vi "borrar.vi"() -> ()   [LabVIEW 2013]
uses:
  <vilib>/Platform/TimedLoop/XDataNode/timing_clust.ctl
  <vilib>/Platform/TimedLoop/XDataNode/nitl_modes.ctl
  <vilib>/Platform/TimedLoop/XDataNode/wakeup.ctl
  <vilib>/addons/database/Connection.llb/DB Tools Open Connec (Path).vi
  <vilib>/platform/TimedLoop/XDataNode/XDataNode.xnode
  <vilib>/addons/database/_DB Variant To Data/Database Variant To Data.xnode
  <vilib>/Platform/TimedLoop/XDataNode/XDNodeRunTimeDep.lvlib
  <vilib>/addons/database/NI_Database_API.lvlib
panel:
  in  "Menu Ring 2":u16(ring) items=["prueba1", "prueba2", "prueba3", "prueba5"]
  in  "Menu Ring":u16(ring) items=["fallo1", "fallo2", "fallo3"]
  out "data 3":string[](array[string])
  out "data 2":string[](array[string])
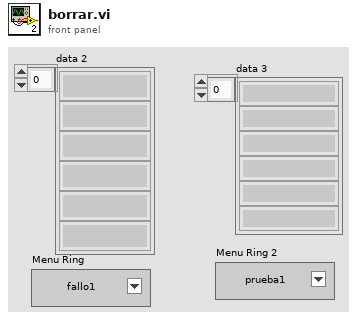
[diagram p1: front panel]
types:
  T1 = typedef "XDNodeRunTimeDep.lvlib/timing_clust.ctl" = cluster{"Expected End [f-1]":u64, "Actual End [f-1]":u64, "Finished Late? [f-1]":bool, "Expected End [i-1]":u64, "Actual End [i-1]":u64, "Finished Late? [i-1]":bool, "Expected Start [i]":u64, "Actual Start [i]":u64, "Expected Start [f]":u64, "Actual Start [f]":u64, "Source Name":string, "Structure Name":string, "Period":i64, "Deadline":i64, "Offset":i64, "Start":i64, "Priority":i32, "Timeout":i32, "Mode":T2, "Wakeup Reason":T3, "Error":errorcluster, "Source Type":string, "Secondary Source Type":string, "Global End Time":u64, "Global Start Time":u64, "Frame Duration":u64, "Iteration Duration":u64, "Assigned CPU":i32, "I/O Scan Engine Mode":u32}
  T2 = typedef "XDNodeRunTimeDep.lvlib/nitl_modes.ctl" = enum32{"No Change", "Process missed periods, maintain original phase", "Discard missed periods, maintain original phase", "Process missed periods, ignore original phase", "Discard missed periods, ignore original phase"}
  T3 = typedef "XDNodeRunTimeDep.lvlib/wakeup.ctl" = enum32{"Normal", "Aborted", "Asynchronous wakeup", "Timing source error", "Timed loop error", "Timeout"}
  T4 = typedef "NI_Database_API.lvlib/Conn ObjectReference.ctl" = refnum<k1>
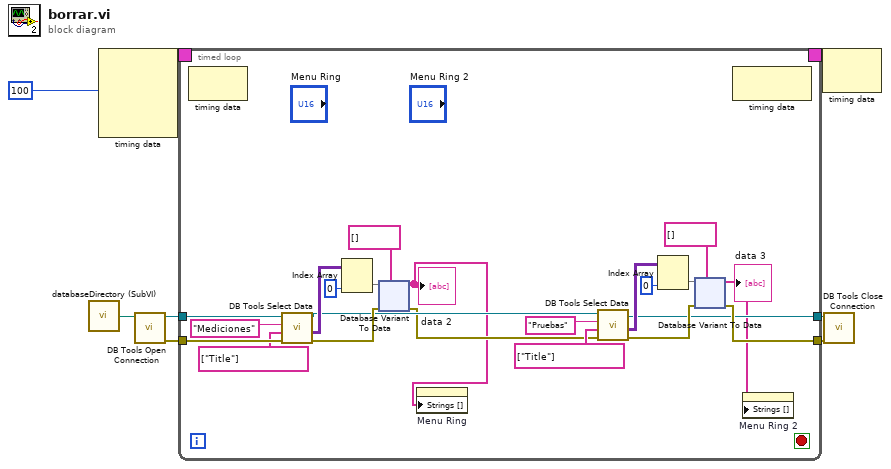
[diagram p0: block diagram]
diagram:
  n1 = call "databaseDirectory (SubVI).vi"() -> ("Application Directory"=w5:path)  [unwired: 1 in]
  n2 = node-c288(i64 100 ("Period")) -> (w8:T1)  [unwired: 3 in]
  n3 = call-poly <vilib>:"DB Tools Open Connection.vi"("connection information"=w5) -> ("error out"=w3:errorcluster, "connection reference"=w4:T4)  [unwired: 7 in]
  n4 = timed-loop {
    timing: w8 -> [_]
    timing-out: [_] -> w7
    tunnel: w4 -> [w30]
    tunnel: w3 -> [w29]
    tunnel: [w12] -> w2
    tunnel: [w11] -> w1
    stop <- _ stop-if-true
    n5 = node-c288() -> ()  [unwired: 1 in, 1 out]
    n6 = call <vilib>:"DB Tools Select Data.vi"("error in (no error)"=w29, "columns"=string[] ["Title"], "table"="Mediciones", "connection reference"=w30) -> ("error out"=w22:errorcluster, "data"=w25:variant[][], "connection reference out"=w14:T4)  [unwired: 2 in]
    n7 = Index Array(array=w25, index (col)=0 ("index")) -> (element=w24:variant[])  [unwired: 1 in]
    n8 = xnode "Database Variant To Data"("database variant"=w24, "error in (no error)"=w22, "type"=string[] []) -> ("data"=w10:string[], "error out"=w13:errorcluster)
    "data 2" <- w10
    n9 = property on="Menu Ring" class="Ring (strict)"("Strings []"=w10) -> ()  [unwired: 2 in, 2 out]
    n10 = call <vilib>:"DB Tools Select Data.vi"("error in (no error)"=w13, "columns"=string[] ["Title"], "table"="Pruebas", "connection reference"=w14) -> ("error out"=w21:errorcluster, "data"=w18:variant[][], "connection reference out"=w11:T4)  [unwired: 2 in]
    n11 = Index Array(array=w18, index (col)=0 ("index")) -> (element=w19:variant[])  [unwired: 1 in]
    n12 = xnode "Database Variant To Data"("database variant"=w19, "error in (no error)"=w21, "type"=string[] []) -> ("data"=w9:string[], "error out"=w12:errorcluster)
    "data 3" <- w9
    n13 = node-c288() -> ()  [unwired: 1 in, 1 out]
    n14 = property on="Menu Ring 2" class="Ring (strict)"("Strings []"=w9) -> ()  [unwired: 2 in, 2 out]
  }
  n15 = node-c288(w7) -> ()  [unwired: 1 out]
  n16 = call <vilib>:"DB Tools Close Connection.vi"("error in (no error)"=w2, "connection reference"=w1) -> ()  [unwired: 5 in, 1 out]
